vi "RichToFlatnixnet_grpc_FrameRequest.vi"(5 "OutputClusterType":T1, 11 "InputCluster":T4) -> (3 "OutputCluster":T1)   [LabVIEW 2025, in "xnet-grpc_client.lvlib"]
uses:
  xnet-grpc_client.lvlib
  nixnet_grpc_FrameRequest.ctl
  nixnet_grpc_FrameRequest_type_enum/nixnet_grpc_FrameRequest_type_enum.lvclass
  nixnet_grpc_FrameFlags.ctl
  nixnet_grpc_FrameRequest_Flat.ctl
  nixnet_grpc_FrameType.ctl
  nixnet_grpc_FrameRequest_type_enum/nixnet_grpc_FrameRequest_type_enum.lvclass/nixnet_grpc_FrameRequest_type_enum.ctl
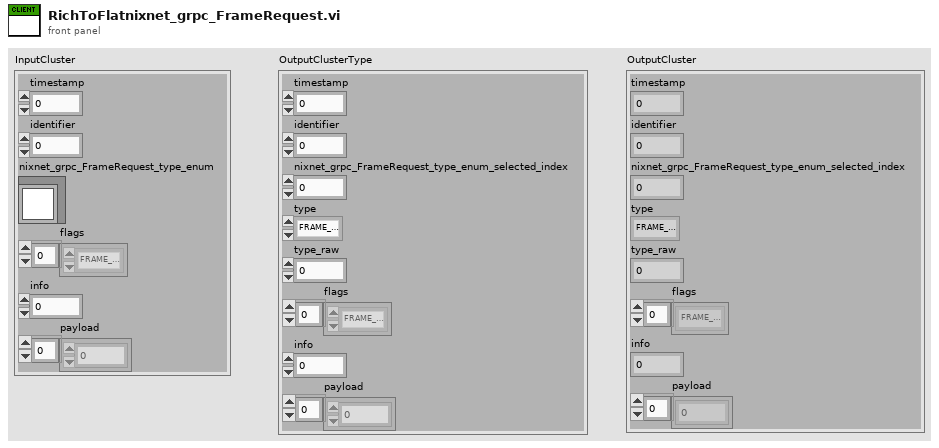
[diagram p1: front panel]
types:
  T1 = typedef "xnet-grpc_client.lvlib/nixnet_grpc_FrameRequest_Flat.ctl" = cluster{"timestamp":u64, "identifier":u32, "nixnet_grpc_FrameRequest_type_enum_selected_index":i32, "type":T2, "type_raw":u32, "flags":T3[], "info":u32, "payload":u8[]}
  T2 = typedef "xnet-grpc_client.lvlib/nixnet_grpc_FrameType.ctl" = enum32{"FRAME_TYPE_CAN_DATA", "FRAME_TYPE_CAN_REMOTE", "FRAME_TYPE_CAN_BUS_ERROR", "FRAME_TYPE_CAN20_DATA", "FRAME_TYPE_CANFD_DATA", "FRAME_TYPE_CANFDBRS_DATA", "FRAME_TYPE_FLEX_RAY_DATA", "FRAME_TYPE_FLEX_RAY_NULL", "FRAME_TYPE_FLEX_RAY_SYMBOL", "FRAME_TYPE_LIN_DATA", "FRAME_TYPE_LIN_BUS_ERROR", "FRAME_TYPE_LIN_NO_RESPONSE", "FRAME_TYPE_J1939_DATA", "FRAME_TYPE_SPECIAL_DELAY", "FRAME_TYPE_SPECIAL_LOG_TRIGGER", "FRAME_TYPE_SPECIAL_START_TRIGGER"}
  T3 = typedef "xnet-grpc_client.lvlib/nixnet_grpc_FrameFlags.ctl" = enum32{"FRAME_FLAGS_UNSPECIFIED", "FRAME_FLAGS_FLEX_RAY_STARTUP", "FRAME_FLAGS_FLEX_RAY_SYNC", "FRAME_FLAGS_FLEX_RAY_PREAMBLE", "FRAME_FLAGS_FLEX_RAY_CH_A", "FRAME_FLAGS_FLEX_RAY_CH_B", "FRAME_FLAGS_LIN_EVENT_SLOT", "FRAME_FLAGS_TRANSMIT_ECHO"}
  T4 = typedef "xnet-grpc_client.lvlib/nixnet_grpc_FrameRequest.ctl" = cluster{"timestamp":u64, "identifier":u32, "nixnet_grpc_FrameRequest_type_enum":refnum<class "nixnet_grpc_FrameRequest_type_enum.lvclass">, "flags":T3[], "info":u32, "payload":u8[]}
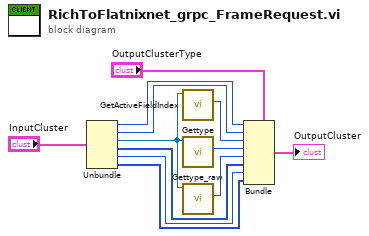
[diagram p0: block diagram]
diagram:
  n1 = Unbundle "Unbundle"("InputCluster") -> ("timestamp"=w9:u64, "identifier"=w8:u32, "nixnet_grpc_FrameRequest_type_enum"=w7:refnum<class "nixnet_grpc_FrameRequest_type_enum.lvclass">, "flags"=w3:T3[], "info"=w2:u32, "payload"=w1:u8[])
  n2 = call "GetActiveFieldIndex.vi"("OneOfTemplate in"=w7) -> ("Active Field Index"=w6:i32)  [unwired: 8 in, 2 out]
  n3 = call "Gettype.vi"("OneOfTemplate in"=w7) -> ("Get_Val"=w5:T2)  [unwired: 8 in, 2 out]
  n4 = call "Gettype_raw.vi"("OneOfTemplate in"=w7) -> ("Get_Val"=w4:u32)  [unwired: 8 in, 2 out]
  n5 = Bundle "Bundle"(cluster="OutputClusterType", "timestamp"=w9, "identifier"=w8, "nixnet_grpc_FrameRequest_type_enum_selected_index"=w6, "type"=w5, "type_raw"=w4, "flags"=w3, "info"=w2, "payload"=w1) -> (→"OutputCluster":T1)
